vi "optogeneticsGenRandomTargets.vi"(2 "max N":i32=100, 3 "min N":i32, 4 "length":i32=10) -> (0 "random indices (string, :)":string, 1 "random indices":i32[](array[numeric]))   [LabVIEW 2017]
uses:
  d50d81f2-ccba-4394-a547-d15724504d6f.vi
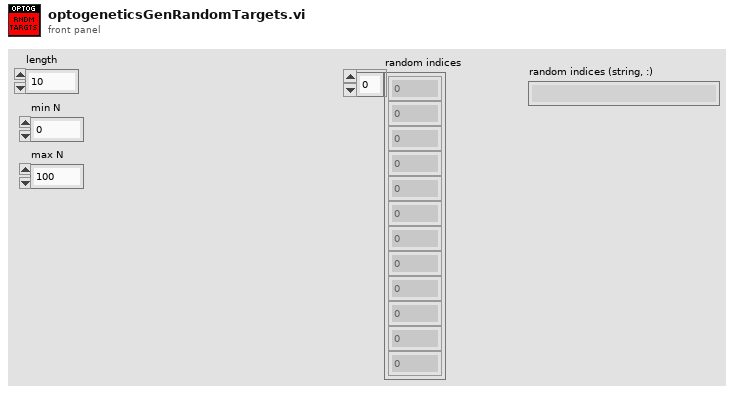
[diagram p1: front panel]
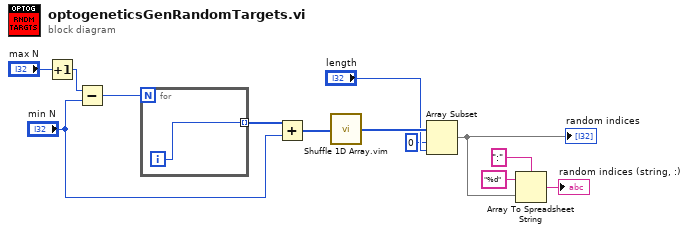
[diagram p0: block diagram]
diagram:
  n1 = Increment(x="max N") -> (x+1=w1:i32)
  n2 = Subtract(x=w1, y="min N") -> (x-y=w12:i32)
  n3 = for {
    N: w12 -> [_]
    tunnel: [w14] -> w11 mode=indexing
    i -> [w14]
  }
  n4 = Add(x=w11, y="min N") -> (x+y=w9:i32[])
  n5 = call "Shuffle 1D Array.vim"("array"=w9) -> ("shuffled array"=w8:i32[])  [unwired: 4 in]
  n6 = Array Subset(array=w8, index=0, length="length") -> (w5:i32[])
  "random indices" <- w5
  n7 = Array To Spreadsheet String(delimiter (Tab)=":", array=w5, 3:"%d" ("format string")) -> (spreadsheet string=→"random indices (string, :)":string)
